vi "Read connects.vi"(8 "error in (no error)":errorcluster, 11 "MBs":refnum<class "Modbus Master CR.lvclass">[](array[class])) -> (0 "error out":errorcluster, 2 "connects":bool[](array[boolean]), 3 "MBs out":refnum<class "Modbus Master CR.lvclass">[](array[class]))   [LabVIEW 2021, in "Modbus Master CR.lvclass"]
uses:
  Modbus Master CR.lvclass
  Modbus Master CR.lvclass/Modbus Master CR.ctl
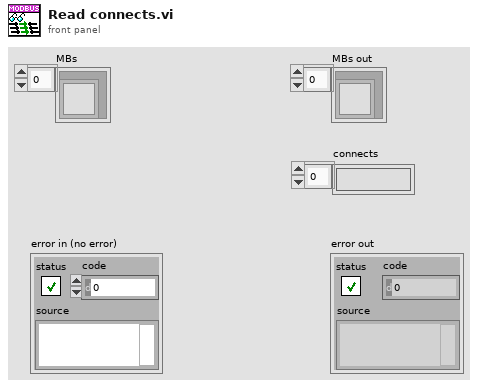
[diagram p1: front panel]
types:
  T1 = typedef "Modbus Master CR.lvclass/MB state.ctl" = cluster{"state":T2, "enable":bool, "Run":bool, "write enable":bool, "Write":bool, "connect":bool, "errors":i32}
  T2 = typedef "MB_v2.lvlib/Modbus Master CR.lvclass/MB_TCP_State.ctl" = enum8{"initialization", "redefine", "standby", "ping", "connect", "wait to reconnect", "wait to reset timeout", "configure", "requests", "close connection", "stop"}
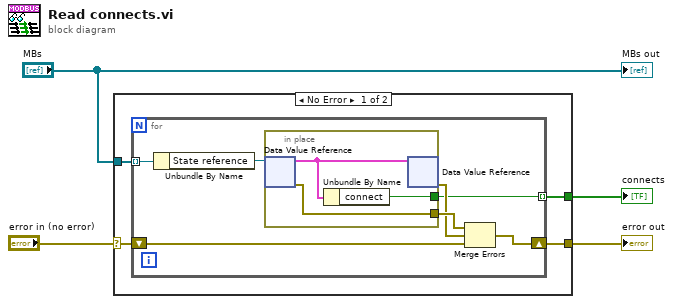
[diagram p0: block diagram]
diagram:
  n1 = case shown="No Error" "error in (no error)" {
    selector: "error in (no error)" -> [w8 w19]
    tunnel: [w7 w19] -> w3
    tunnel: "MBs" -> [w5 _]
    tunnel: [w6 _] -> w1
    frame No Error {
      n2 = for {
        tunnel: [w10] -> w6 mode=indexing
        tunnel: w5 -> [w9] mode=indexing
        shift-right: [w11] -> w7
        shift-left: w8 -> [w12]
        n3 = Unbundle By Name(w9) -> ("State reference"=w15:refnum<data-value>)
        n4 = in-place {
          in-place-border: [w18] -> w14
          in-place-border: [w17] -> w10
          n5 = in-place-dvr #1(w15) -> (w16:T1, w18:errorcluster)
          n6 = Unbundle By Name(w16) -> ("connect"=w17:bool)
          n7 = in-place-dvr #1(w16) -> (w13:errorcluster)  [unwired: 1 out]
        }
        n8 = Merge Errors(w14, w13, w12) -> (w11:errorcluster)
      }
    }
    frame Error {
    }
  }
  "error out" <- w3
  "connects" <- w1
  "MBs out" <- "MBs"
